vi "20211029_04.vi"() -> ()   [LabVIEW 2019]
panel:
  out "Selected Item":string[](array[string])
  in  "Multicolumn Listbox":i32(listbox)
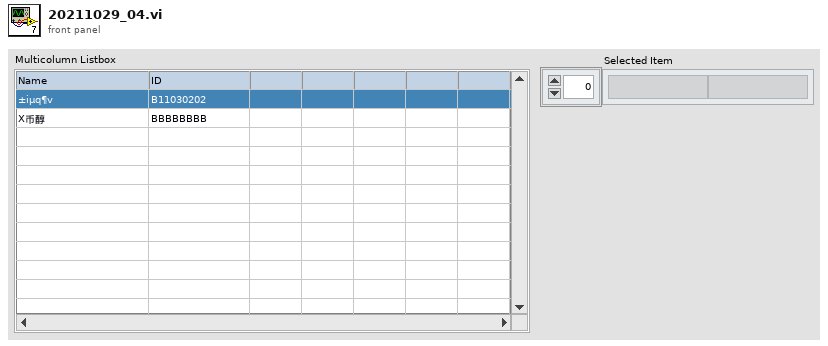
[diagram p1: front panel]
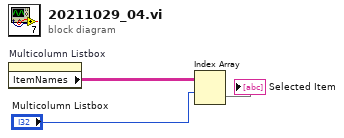
[diagram p0: block diagram]
diagram:
  n1 = property on="Multicolumn Listbox" class="MCListbox (strict)"() -> ("ItemNames"=w3:string[][])  [unwired: 2 in, 2 out]
  n2 = Index Array(array=w3, index (row)="Multicolumn Listbox") -> (element=→"Selected Item":string[])  [unwired: 1 in]
